vi "Append Status Message.vi"(0 "Str Refnum":refnum<vi>, 7 "Message":string, 11 "error in (no error)":errorcluster) -> (15 "error out":errorcluster)   [LabVIEW 2016]
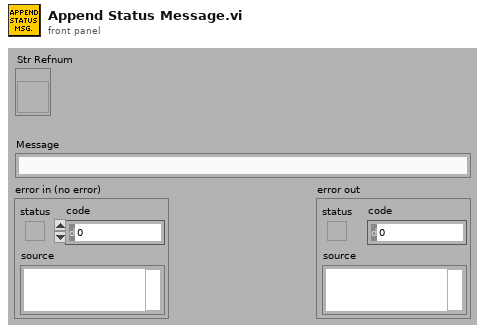
[diagram p1: front panel]
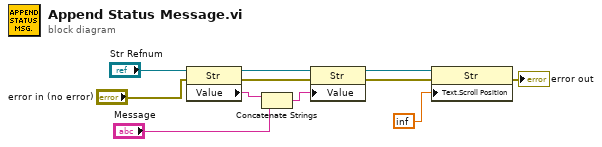
[diagram p0: block diagram]
diagram:
  n1 = property class="Str"(reference="Str Refnum", error in="error in (no error)") -> (reference out=w10:refnum<vi>, error out=w9:errorcluster, "Value"=w8:string)
  n2 = Concatenate Strings(w8, "Message") -> (w7:string)
  n3 = property class="Str"(reference=w10, error in=w9, "Value"=w7) -> (reference out=w4:refnum<vi>, error out=w3:errorcluster)
  n4 = property class="Str"(reference=w4, error in=w3, "Text.Scroll Position"=inf) -> (error out=→"error out":errorcluster)  [unwired: 1 out]
